vi "get_component_type_name.vi"(8 "error in (no error)":errorcluster, 11 "GenericPlugin in":refnum<class "GenericAnalogOut.lvclass">) -> (0 "error out":errorcluster, 2 "component type":string, 3 "GenericPlugin out":refnum<class "GenericAnalogOut.lvclass">)   [LabVIEW 2010, in "GenericAnalogOut.lvclass"]
uses:
  GenericAnalogOut.lvclass
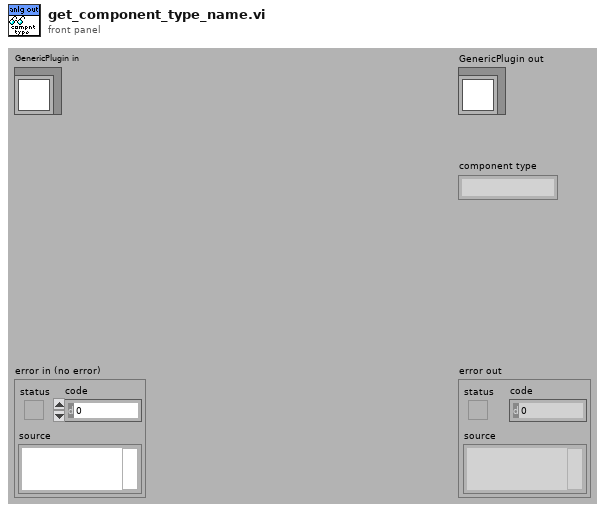
[diagram p1: front panel]
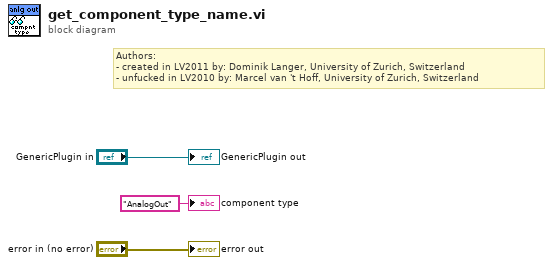
[diagram p0: block diagram]
diagram:
  # "Authors: \n- created in LV2011 by: Dominik Langer, University of Zurich, Switzerland\n- unfucked in LV2010 by: Marcel van 't Hoff, University of Zurich, Switzerland"
  "error out" <- "error in (no error)"
  "GenericPlugin out" <- "GenericPlugin in"
  "component type" <- "AnalogOut" ("component type")
